vi "RC Enum to RC Object.vi"(1 "RC Type":T1) -> (0 "RemoteControl out":refnum<class "RemoteControl.lvclass">)   [LabVIEW 2019, in "RemoteControl.lvclass"]
uses:
  RemoteControl.lvclass
  Typedefs/RC Com Type--enum.ctl
  RemoteControl.ZMQ/RemoteControl.ZMQ.lvclass
  \\Mac\Home/Documents/GitHub/Instrument-Framework/lvsrc/SMOs/RemoteControl/RemoteControl.lvclass
  RemoteControl.STM/RemoteControl.STM.lvclass
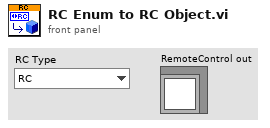
[diagram p1: front panel]
types:
  T1 = typedef "RemoteControl.lvclass/RC Com Type--enum.ctl" = enum16{"RC", "STM", "ZMQ"}
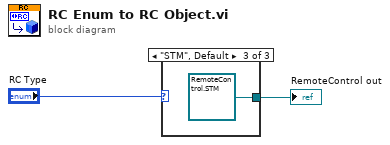
[diagram p0: block diagram]
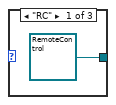
[diagram p2: hidden frame]
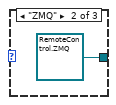
[diagram p3: hidden frame]
diagram:
  n1 = case shown="\"STM\", Default" "RC Type" {
    tunnel: [refnum<class "RemoteControl.lvclass"> refnum ("RemoteControl in") refnum<class "RemoteControl.ZMQ.lvclass"> refnum ("RemoteControl.ZMQ.lvclass") refnum<class "RemoteControl.STM.lvclass"> refnum ("RemoteControl.STM.lvclass")] -> w1
    frame "RC" {
    }
    frame "ZMQ" {
    }
    frame "STM", Default {
    }
  }
  "RemoteControl out" <- w1
